vi "Close.vi"(8 "error in (no error)":errorcluster, 11 "NI Thermo in":refnum<class "NI Thermo.lvclass">) -> (0 "error out":errorcluster, 3 "NI Thermo out":refnum<class "NI Thermo.lvclass">)   [LabVIEW 2025, in "Thermo.lvlib" / "NI Thermo.lvclass"]
uses:
  NI Thermo.lvclass
  NI Thermo.lvclass/NI Thermo.ctl
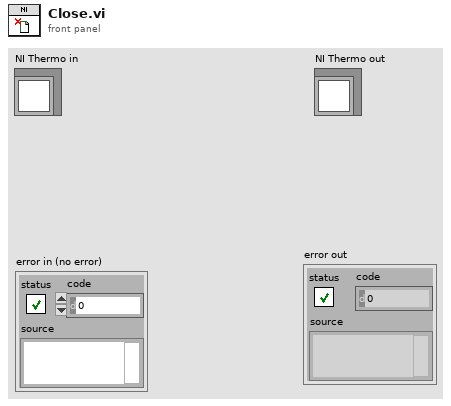
[diagram p1: front panel]
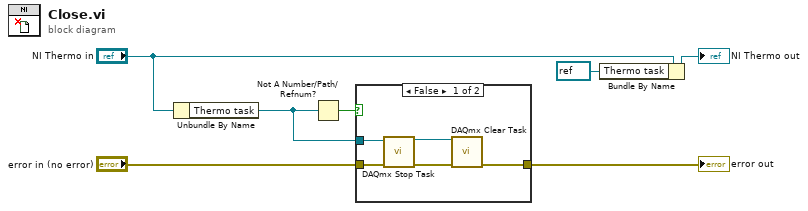
[diagram p0: block diagram]
diagram:
  n1 = Unbundle By Name("NI Thermo in") -> ("Thermo task"=w3:refnum<k21>)
  n2 = Not A Number/Path/Refnum?(number/path/refnum=w3) -> (NaN/Path/Refnum?=w4:bool)
  n3 = case shown="False" w4 {
    tunnel: "error in (no error)" -> [w11 w13]
    tunnel: [w10 w13] -> w5
    tunnel: w3 -> [w9 _]
    frame False {
      n4 = call <vilib>:"DAQmx Stop Task.vi"("task/channels in"=w9, "error in"=w11) -> ("task out"=w8:refnum<k21>, "error out"=w12:errorcluster)  [unwired: 12 in]
      n5 = call <vilib>:"DAQmx Clear Task.vi"("task in"=w8, "error in"=w12) -> ("error out"=w10:errorcluster)  [unwired: 13 in]
    }
    frame True {
    }
  }
  "error out" <- w5
  n6 = Bundle By Name(cluster="NI Thermo in", "Thermo task"=refnum<k21> refnum) -> (→"NI Thermo out":refnum<class "NI Thermo.lvclass">)
